vi "GeneratePredefinedWhiteNoise.vi"(11 "Main Switch":bool) -> (3 "Elapsed Time (s)":dbl format="%#_2f")   [LabVIEW 2022 SP3]
uses:
  <vilib>/sound2/lvsound2.llb/Sound Data Format.ctl
  <vilib>/sound2/lvsound2.llb/Sampling Mode.ctl
  <vilib>/Analysis/4window.llb/windowTd.ctl
  <vilib>/sound2/lvsound2.llb/Sound Output Set Volume (Single).vi
  <vilib>/measure/maspectr.llb/FFT Spectrum (Mag-Phase) for 1 Chan.vi
  <vilib>/measure/matone.llb/Extract Single Tone Information 1 Chan.vi
  <vilib>/sound2/lvsound2.llb/Sound Output Write (DBL Single).vi
  <vilib>/measure/NI_MAPro.lvlib
  <vilib>/Analysis/NI_AALPro.lvlib
panel:
  out "detected amplitude":dbl format="%.2p"
  out "detected frequency":dbl format="%.2p"
  out "FFT":cluster{"f0":dbl, "df":dbl, "magnitude":dbl[]}(graph)
  out "error out":errorcluster
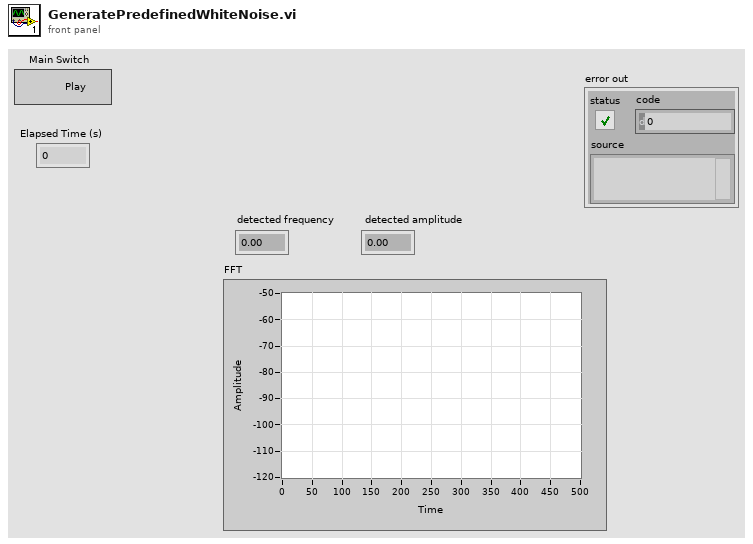
[diagram p1: front panel]
types:
  T1 = typedef "Sound Data Format.ctl" = cluster{"sample rate (S/s)":dbl, "number of channels":i32, "bits per sample":i32}
  T2 = typedef "Sampling Mode.ctl" = i32
  T3 = typedef "Sound Output Task ID.ctl" = u32
  T4 = cluster{"averaging mode":enum16{"No averaging", "Vector averaging", "RMS averaging", "Peak hold"}, "weighting mode":enum16{"Linear", "Exponential"}, "number of averages":u32}
  T5 = cluster{"dB On (F)":bool, "unwrap phase (F)":bool, "convert to degree (F)":bool}
  T6 = typedef "NI_AALPro.lvlib/windowTd.ctl" = u32
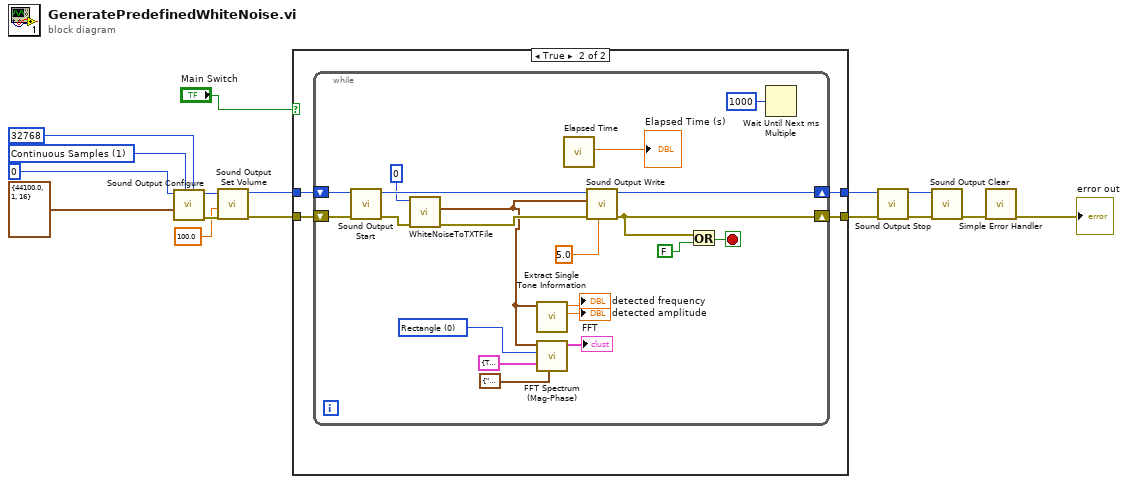
[diagram p0: block diagram]
diagram:
  w12 = T2 1 items=["Finite Samples", "Continuous Samples"] ("sample mode")
  n1 = call <vilib>:"Sound Output Configure.vi"("number of samples/ch"=32768 ("Number of Samples/ch"), "sample mode"=w12, "sound format"=T1 {"sample rate (S/s)"=44100.0, "number of channels"=1, "bits per sample"=16} ("Sound Format"), "device ID"=u32 0 ("Device ID")) -> ("error out"=w15:errorcluster, "task ID"=w16:T3)  [unwired: 6 in]
  n2 = call-poly <vilib>:"Sound Output Set Volume.vi"("error in (no error)"=w15, "volume"=100.0, "task ID"=w16) -> ("error out"=w9:errorcluster, "task ID out"=w8:T3)  [unwired: 7 in]
  n3 = case shown="True" "Main Switch" {
    tunnel: w9 -> [w17 w22]
    tunnel: w8 -> [w18 w21]
    tunnel: [w18 w20] -> w4
    tunnel: [w17 w19] -> w2
    frame False {
    }
    frame True {
      n4 = while {
        shift-right: [w37] -> w20
        shift-left: w21 -> [w38]
        shift-right: [w36] -> w19
        shift-left: w22 -> [w39]
        stop <- w41 stop-if-true
        w26 = T6 0 items=["Rectangle"=0, "Hanning"=1, "Hamming"=2, "Blackman-Harris"=3, "Exact Blackman"=4, "Blackman"=5, "Flat Top"=6, "4 Term B-Harris "=7, "7 Term B-Harris"=8, "Low Sidelobe"=9, "Blackman Nuttall"=11, "Triangle"=30, "Bartlett-Hanning"=31, "Bohman"=32, "Parzen"=33, "Welch"=34, "Kaiser"=60, "Dolph-Chebyshev"=61, "Gaussian"=62] ("window")
        n5 = call <vilib>:"Sound Output Start.vi"("error in (no error)"=w39, "task ID"=w38) -> ("error out"=w33:errorcluster, "task ID out"=w34:T3)  [unwired: 8 in]
        n6 = call "WhiteNoiseToTXTFile.vi"("error in"=w33, "index"=0 ("y")) -> ("error out"=w35:errorcluster, "output waveform"=w24:waveform(dbl))  [unwired: 8 in]
        n7 = call-poly <vilib>:"Extract Single Tone Information.vi"("time signal in"=w24) -> ("detected amplitude"=→"detected amplitude":dbl, "detected frequency"=→"detected frequency":dbl)  [unwired: 5 in, 4 out]
        n8 = call-poly <vilib>:"FFT Spectrum (Mag-Phase).vi"("averaging parameters"=T4 {"averaging mode"=enum."Vector averaging", "weighting mode"=enum."Linear", "number of averages"=10}, "view"=T5 {"dB On (F)"=TRUE, "unwrap phase (F)"=FALSE, "convert to degree (F)"=FALSE}, "window"=w26, "time signal"=w24) -> ("magnitude"=→"FFT":cluster{"f0":dbl, "df":dbl, "magnitude":dbl[]})  [unwired: 3 in, 4 out]
        n9 = call "Elapsed Time"() -> ("Elapsed Time (s)"=→"Elapsed Time (s)":dbl)  [unwired: 12 in, 7 out]
        n10 = call-poly <vilib>:"Sound Output Write.vi"("timeout (sec)"=5.0, "error in (no error)"=w35, "data"=w24, "task ID"=w34) -> ("error out"=w36:errorcluster, "task ID out"=w37:T3)  [unwired: 6 in]
        n11 = Or(x=w36, y=FALSE ("End Execution")) -> (x .or. y?=w41:bool)
        n12 = Wait Until Next ms Multiple(millisecond multiple=u32 1000) -> ()  [unwired: 1 out]
      }
    }
  }
  n13 = call <vilib>:"Sound Output Stop.vi"("error in (no error)"=w2, "task ID"=w4) -> ("error out"=w6:errorcluster, "task ID out"=w7:T3)  [unwired: 8 in]
  n14 = call <vilib>:"Sound Output Clear.vi"("error in (no error)"=w6, "task ID"=w7) -> ("error out"=w5:errorcluster)  [unwired: 9 in]
  n15 = call <vilib>:"Simple Error Handler.vi"("error in (no error)"=w5) -> ("error out"=→"error out":errorcluster)  [unwired: 4 in, 4 out]
